vi "LVProjectShortcut_CreateNewWizard_Interface.vi"() -> (3 "InterfaceTable":T1)   [LabVIEW 2017, in "LVProject Shortcut.lvlib"]
doc: "NI Confidential \n\n/**\n@brief This VI tells the framework which VIs to call when an event happens related to one of your items.\n\n@author Joel Dixon\n\n@par Sample_Item_Interface.vi\n For each of the entries in the InterfaceTable, pass in a string representing a relative path to a VI which implements that method. Methods include Init, Exit, OnCommand, OnDropFiles, and OnSelect. \n\n@param \"InterfaceTable\" [out] \nThis is an array of strings passed back to the framework so it knows which VIs should be called under what circumstances.\n*/"
uses:
  <resource>/Framework/Providers/API/CreateNewWizard_Interface.ctl
  LVProject Shortcut.lvlib
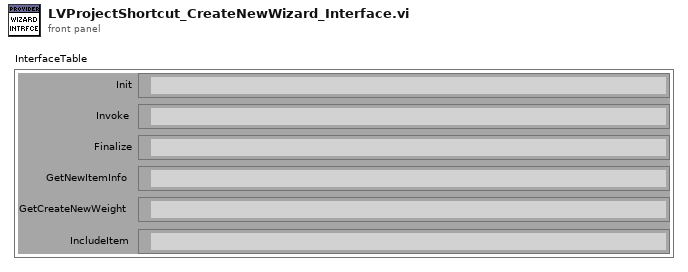
[diagram p1: front panel]
types:
  T1 = typedef "CreateNewWizard_Interface.ctl" = cluster{"Init":path, "Invoke":path, "Finalize":path, "GetNewItemInfo":path, "GetCreateNewWeight":path, "IncludeItem":path}
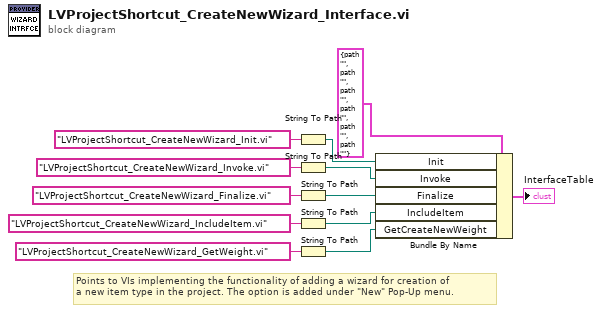
[diagram p0: block diagram]
diagram:
  # "Points to VIs implementing the functionality of adding a wizard for creation of \na new item type in the project. The option is added under \"New\" Pop-Up menu."
  n1 = String To Path(string="LVProjectShortcut_CreateNewWizard_Init.vi" ("vi path")) -> (path=w10:path)
  n2 = String To Path(string="LVProjectShortcut_CreateNewWizard_Invoke.vi" ("vi path")) -> (path=w9:path)
  n3 = String To Path(string="LVProjectShortcut_CreateNewWizard_Finalize.vi" ("vi path")) -> (path=w8:path)
  n4 = String To Path(string="LVProjectShortcut_CreateNewWizard_IncludeItem.vi") -> (path=w4:path)
  n5 = String To Path(string="LVProjectShortcut_CreateNewWizard_GetWeight.vi") -> (path=w1:path)
  n6 = Bundle By Name(cluster=T1 {"Init"=path "", "Invoke"=path "", "Finalize"=path "", "GetNewItemInfo"=path "", "GetCreateNewWeight"=path "", "IncludeItem"=path ""} ("InterfaceTable"), "Init"=w10, "Invoke"=w9, "Finalize"=w8, "IncludeItem"=w4, "GetCreateNewWeight"=w1) -> (→"InterfaceTable":T1)
